vi "F Dwf Analog In Sampling Source Get.vi"(8 "error in (no error)":errorcluster, 10 "ptrigsrc":string, 11 "hdwf":i32) -> (0 "error out":errorcluster, 2 "ptrigsrc out":string, 3 "function return":i32)   [LabVIEW 2019, in "Olasdwf.lvlib"]
doc: "DWFAPI int FDwfAnalogInSamplingSourceGet(HDWF hdwf, TRIGSRC *ptrigsrc);"
uses:
  Olasdwf.lvlib
  Windows/System32/dwf.dll
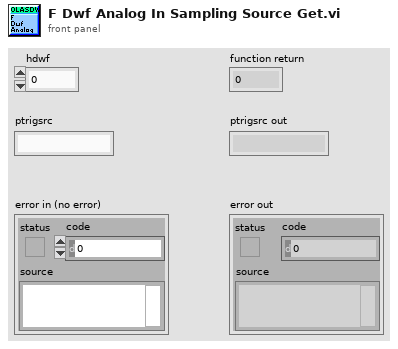
[diagram p1: front panel]
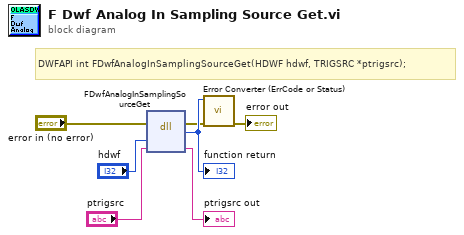
[diagram p0: block diagram]
diagram:
  # "DWFAPI int FDwfAnalogInSamplingSourceGet(HDWF hdwf, TRIGSRC *ptrigsrc);"
  n1 = dll-call lib="C:/Windows/System32/dwf.*" fn="FDwfAnalogInSamplingSourceGet"(error in="error in (no error)", "hdwf"="hdwf", "ptrigsrc"="ptrigsrc") -> (error out=w2:errorcluster, w7:i32, "ptrigsrc"=→"ptrigsrc out":string)  [unwired: 3 in, 1 out]
  "function return" <- w7
  n2 = call "Error Converter (ErrCode or Status).vi"("error in (no error)"=w2, "error code"=w7) -> ("error out"=→"error out":errorcluster)  [unwired: 9 in]
